vi "test_timeout condition.vi"(8 "error in (no error)":errorcluster, 11 "TestCase in":refnum<class "Return Response Triggers.lvclass">) -> (0 "error out":errorcluster, 3 "TestCase out":refnum<class "Return Response Triggers.lvclass">)   [LabVIEW 2017, in "Return Response Triggers.lvclass"]
uses:
  Return Response Triggers.lvclass
  Libraries/SSH/Return Request Configuration.ctl
  Libraries/SSH/Response Configuration.ctl
  fb912344-4e5e-41e8-af55-9ce47520e721.vi
  <vilib>/addons/_JKI Toolkits/VI Tester/TestCase.llb/TestCase.lvclass
  Libraries/SSH/SSH.lvlib
  C:/Program Files (x86)/National Instruments/LabVIEW 2017/vi.lib/addons/_JKI Toolkits/VI Tester/TestCase.llb/TestCase.lvclass
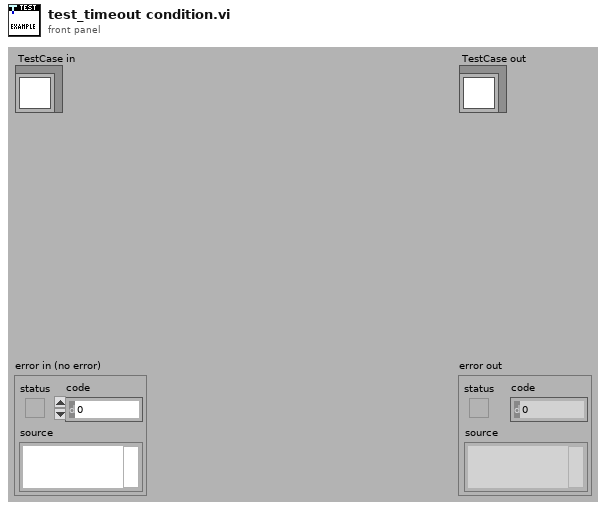
[diagram p1: front panel]
types:
  T1 = typedef "SSH.lvlib/Return Request Configuration.ctl" = cluster{"Response Configuration":T2, "Return Notifier":refnum<notifier>, "Response Requested":bool, "Command":string, "Initial Timer Value":u32}
  T2 = typedef "SSH.lvlib/Response Configuration.ctl" = cluster{"Expected Response":string, "Character Count Limit":i32, "Timeout (ms)":i32}
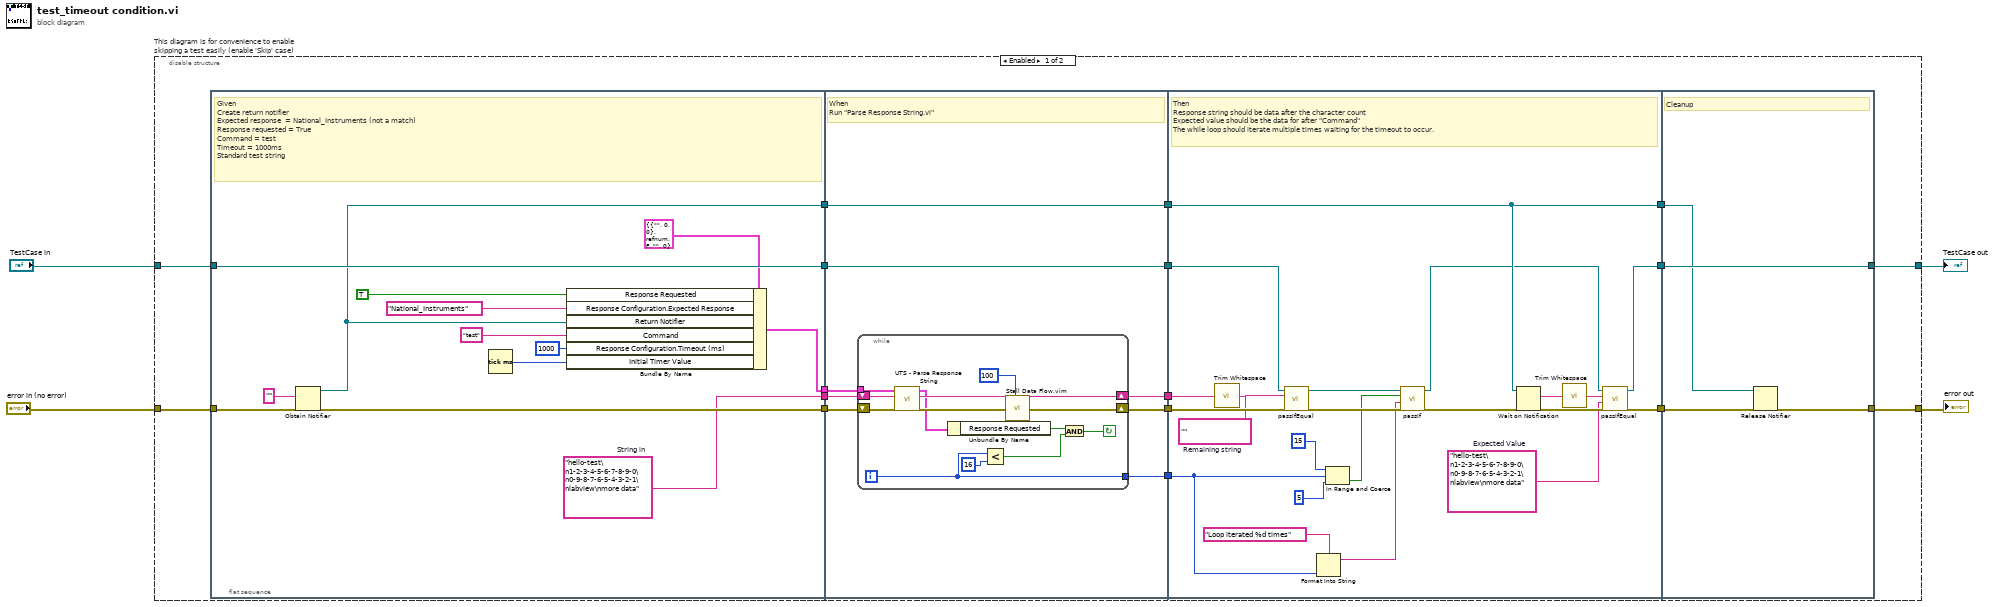
[diagram p0: block diagram]
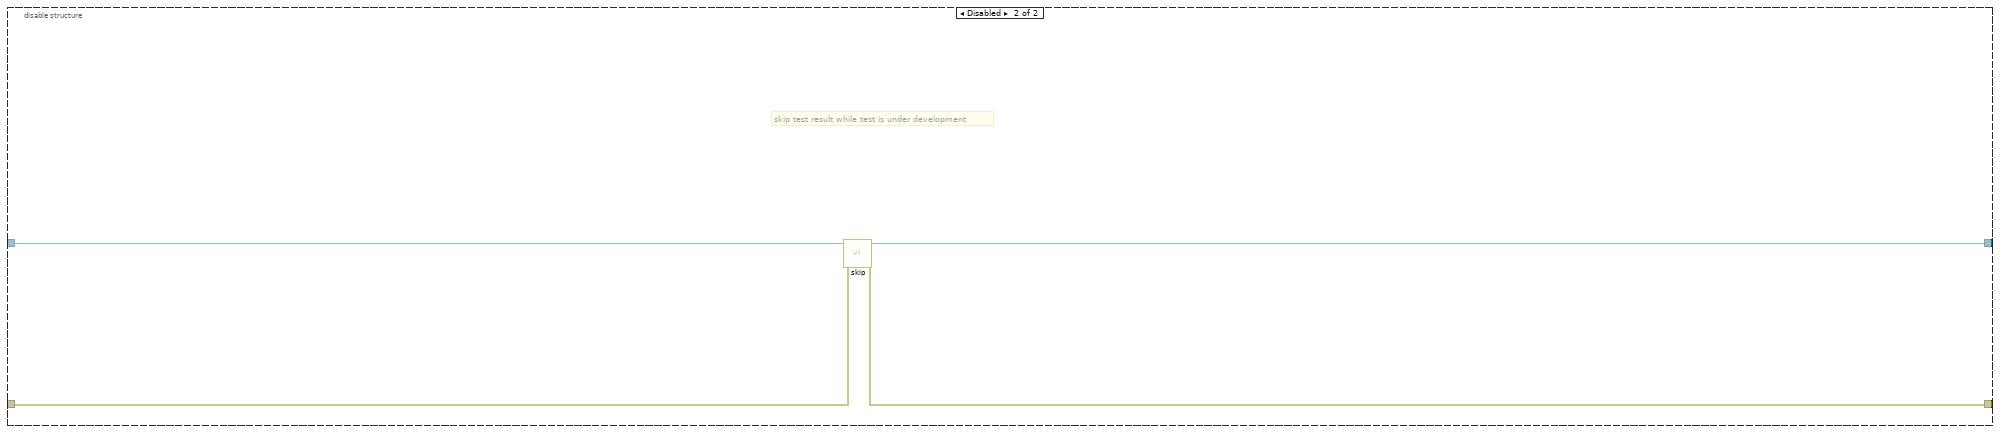
[diagram p2: hidden frame]
diagram:
  n1 = disable-structure "This diagram is for convenience to enable skipping a test easily (enable 'Skip' case)" shown="Enabled" {
    disable-tunnel: "TestCase in" -> [w14 w85]
    disable-tunnel: [w13 w83] -> w1
    disable-tunnel: [w12 w84] -> w3
    disable-tunnel: "error in (no error)" -> [w15 w82]
    frame Enabled {
      n2 = flat-sequence {
        tunnel: w15 -> [w31]
        tunnel: w14 -> [w34]
        tunnel: [w34] -> w21
        tunnel: [w30] -> w20
        tunnel: [w29] -> w11
        tunnel: [w25] -> w10
        tunnel: [w24] -> w9
        tunnel: [w42] -> w19
        tunnel: [w40] -> w18
        tunnel: w21 -> [w42]
        tunnel: w20 -> [w41]
        tunnel: w11 -> [w39]
        tunnel: w10 -> [w36]
        tunnel: w9 -> [w38]
        tunnel: [w37] -> w8
        tunnel: [w36] -> w7
        tunnel: [w35] -> w5
        tunnel: [w71] -> w17
        tunnel: [w72] -> w16
        tunnel: w19 -> [w77]
        tunnel: w18 -> [w76]
        tunnel: w8 -> [w74]
        tunnel: w7 -> [w68]
        tunnel: [w68] -> w6
        tunnel: w5 -> [w57]
        tunnel: [w79] -> w12
        tunnel: [w81] -> w13
        tunnel: w17 -> [w81]
        tunnel: w16 -> [w80]
        tunnel: w6 -> [w78]
        frame #0 {
          w24 = "hello-test\n1-2-3-4-5-6-7-8-9-0\n0-9-8-7-6-5-4-3-2-1\nlabview\nmore data"  # String in
          # "Given\nCreate return notifier\nExpected response  = National_Instruments (not a match)\nResponse requested = True\nCommand = test\nTimeout = 1000ms\nStandard test string"
          n3 = Obtain Notifier(notification data type="", error in (no error)=w31) -> (notifier out=w25:refnum<notifier>, error out=w30:errorcluster)  [unwired: 2 in, 1 out]
          n4 = Tick Count (ms)() -> (millisecond timer value=w22:u32)
          n5 = Bundle By Name(cluster=T1 {"Response Configuration"={"Expected Response"="", "Character Count Limit"=0, "Timeout (ms)"=0}, "Return Notifier"=refnum, "Response Requested"=FALSE, "Command"="", "Initial Timer Value"=0} ("Return Request in"), "Response Requested"=TRUE, "Response Configuration.Expected Response"="National_Instruments", "Return Notifier"=w25, "Command"="test", "Response Configuration.Timeout (ms)"=u32 1000, "Initial Timer Value"=w22) -> (w29:T1)
        }
        frame #1 {
          # "When\nRun \"Parse Response String.vi\""
          n6 = while {
            tunnel: w39 -> [w53]
            shift-right: [w49] -> w40
            shift-left: w41 -> [w55]
            shift-right: [w51] -> w37
            shift-left: w38 -> [w52]
            tunnel: [w47] -> w35
            i -> [w47]
            stop <- w43 continue-if-true
            n7 = call "UTS - Parse Response String.vi"("error in (no error)"=w55, "Response String in"=w52, "Return Request in"=w53) -> ("error out"=w54:errorcluster, "Response String out"=w51:string, "Return Request out"=w50:T1)  [unwired: 6 in]
            n8 = Unbundle By Name(w50) -> ("Response Requested"=w45:bool)
            n9 = Less?(x=w47, y=16) -> (x < y?=w44:bool)
            n10 = call "Stall Data Flow.vim"("value in"=w54, "milliseconds to wait"=u32 100) -> ("value out"=w49:errorcluster)  [unwired: 1 out]
            n11 = And(x=w45, y=w44) -> (x .and. y?=w43:bool)
          }
        }
        frame #2 {
          w67 = ""  # Remaining string
          w70 = "hello-test\n1-2-3-4-5-6-7-8-9-0\n0-9-8-7-6-5-4-3-2-1\nlabview\nmore data"  # Expected Value
          # "Then\nResponse string should be data after the character count\nExpected value should be the data for after \"Command\"\nThe while loop should iterate multiple times waiting for the timeout to occur."
          n12 = call <vilib>:"Trim Whitespace.vi"("string"=w74) -> ("trimmed string"=w66:string)  [unwired: 1 in]
          n13 = call-dynamic "passIfEqual.vi"("error in (no error)"=w76, "y"=w67, "x"=w66, "TestCase in"=w77) -> ("error out"=w75:errorcluster, "TestCase out"=w61:refnum<class "Return Response Triggers.lvclass">)  [unwired: 6 in]
          n14 = Format Into String(format string="Loop iterated %d times", w57) -> (resulting string=w58:string)  [unwired: 2 in, 1 out]
          n15 = In Range and Coerce(upper limit=15, x=w57, lower limit=5 ("y")) -> (In Range?=w62:bool)  [unwired: 1 out]
          n16 = call-dynamic "passIf.vi"("error in (no error)"=w75, "message (\"\")"=w58, "pass"=w62, "TestCase in"=w61) -> ("error out"=w64:errorcluster, "TestCase out"=w60:refnum<class "Return Response Triggers.lvclass">)  [unwired: 6 in]
          n17 = Wait on Notification(notifier=w68, error in (no error)=w64) -> (notification=w69:string, error out=w73:errorcluster)  [unwired: 2 in, 2 out]
          n18 = call <vilib>:"Trim Whitespace.vi"("string"=w69) -> ("trimmed string"=w65:string)  [unwired: 1 in]
          n19 = call-dynamic "passIfEqual.vi"("error in (no error)"=w73, "y"=w70, "x"=w65, "TestCase in"=w60) -> ("error out"=w72:errorcluster, "TestCase out"=w71:refnum<class "Return Response Triggers.lvclass">)  [unwired: 6 in]
        }
        frame #3 {
          # "Cleanup"
          n20 = Release Notifier(notifier=w78, error in (no error)=w80) -> (error out=w79:errorcluster)  [unwired: 1 in, 2 out]
        }
      }
    }
    frame Disabled {
      # "skip test result while test is under development"
      n21 = call <vilib>:"skip.vi"("error in (no error)"=w82, "TestCase in"=w85) -> ("error out"=w84:errorcluster, "TestCase out"=w83:refnum<class "Return Response Triggers.lvclass">)  [unwired: 8 in]
    }
  }
  "error out" <- w3
  "TestCase out" <- w1
